vi "AlliGator Enter Reference Lifetime Dialog.vi"(8 "Error In":errorcluster, 11 "Input Message":string="Enter phase lifetime to use as refrence:") -> (0 "Error Out":errorcluster, 1 "Cancelled?":bool, 3 "Reference Lifetime":dbl[unit])   [LabVIEW 2021, in "AlliGator Phasor Graph.lvlib"]
doc: "Reference Lifetime dialog."
uses:
  AlliGator Phasor Graph.lvlib
panel:
  in  "Reference Lifetime":dbl[unit] min=0.0 format="%.3g"
  in  "Cancel":bool
  in  "OK":bool
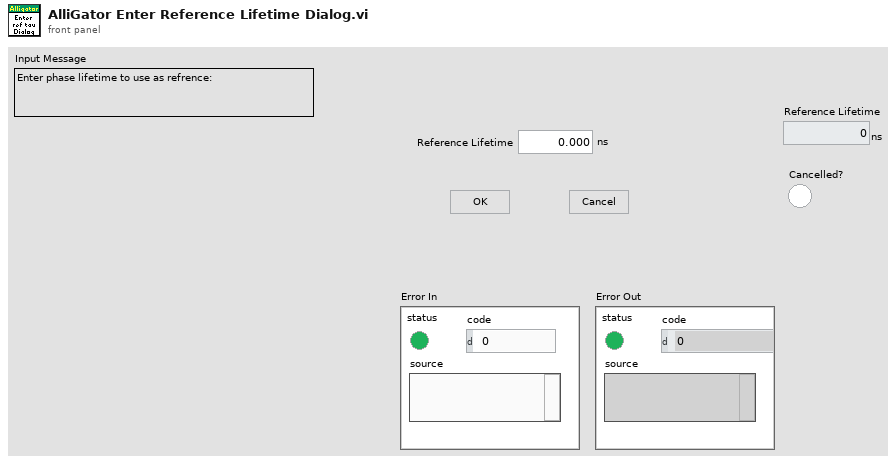
[diagram p1: front panel]
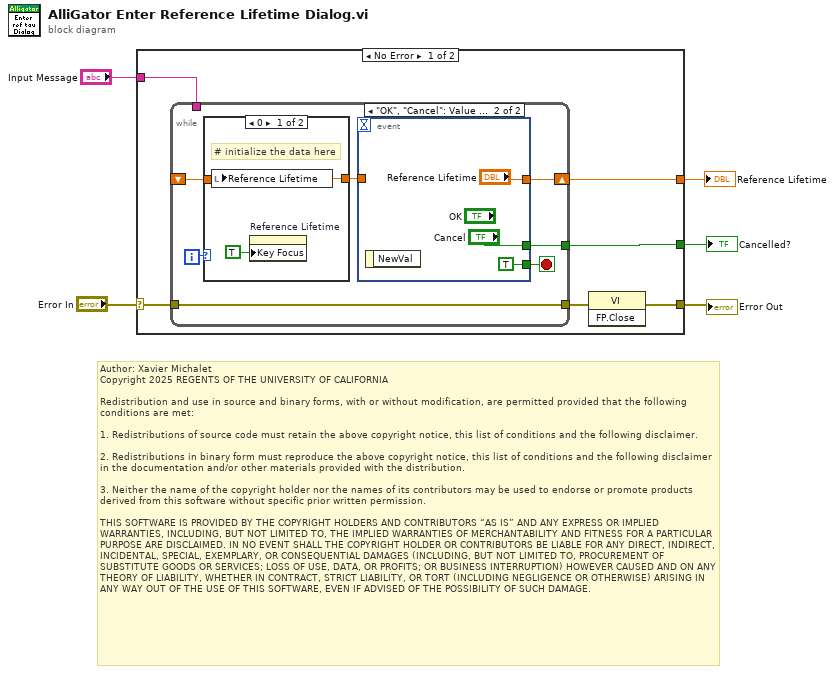
[diagram p0: block diagram]
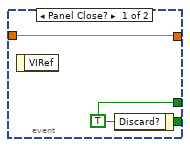
[diagram p3: hidden frame]
diagram:
  # "Author: Xavier Michalet\nCopyright 2025 REGENTS OF THE UNIVERSITY OF CALIFORNIA\n\nRedistribution and use in source and binary forms, with or without modification, are permitted provided that the following conditions are met:\n\n1. Redistributions of source code must retain the above copyright notice, this list of conditions and the following disclaimer.\n\n2. Redistributions in binary form must reproduce the above copyright notice, this list of conditions and the following disclaimer in the documentation and/or other materials provided with the distribution.\n\n3. Neither the name of the copyright holder nor the names of its contributors may be used to endorse or promote products derived from this software without specific prior written permission.\n\nTHIS SOFTWARE IS PROVIDED BY THE COPYRIGHT HOLDERS AND CONTRIBUTORS “AS IS” AND ANY EXPRESS OR IMPLIED WARRANTIES, INCLUDING, BUT NOT LIMITED TO, THE IMPLIED WARRANTIES OF MERCHANTABILITY AND FITNESS FOR A PARTICULAR PURPOSE ARE DISCLAIMED. IN NO EVENT SHALL THE COPYRIGHT HOLDER OR CONTRIBUTORS BE LIABLE FOR ANY DIRECT, INDIRECT, INCIDENTAL, SPECIAL, EXEMPLARY, OR CONSEQUENTIAL DAMAGES (INCLUDING, BUT NOT LIMITED TO, PROCUREMENT OF SUBSTITUTE GOODS OR SERVICES; LOSS OF USE, DATA, OR PROFITS; OR BUSINESS INTERRUPTION) HOWEVER CAUSED AND ON ANY THEORY OF LIABILITY, WHETHER IN CONTRACT, STRICT LIABILITY, OR TORT (INCLUDING NEGLIGENCE OR OTHERWISE) ARISING IN ANY WAY OUT OF THE USE OF THIS SOFTWARE, EVEN IF ADVISED OF THE POSSIBILITY OF SUCH DAMAGE."
  n1 = case shown="No Error" "Error In" {
    selector: "Error In" -> [w7 w27]
    tunnel: [w11 _] -> w5
    tunnel: [w10 _] -> w4
    tunnel: "Input Message" -> [w9 _]
    tunnel: [w8 w27] -> w1
    frame No Error {
      n2 = while {
        tunnel: [w17] -> w11
        shift-right: [w14] -> w10
        shift-left: _ -> [w15]
        tunnel: w9 -> [_]
        tunnel: w7 -> [w12]
        tunnel: [w12] -> w6
        i -> [w16]
        stop <- w18 stop-if-true
        n3 = case shown="0" w16 {
          tunnel: w15 -> [w20 w21]
          tunnel: [w20 w21] -> w13
          frame 0 {
            # "# initialize the data here"
            n4 = local write "Reference Lifetime"(w20) -> ()
            n5 = property on="Reference Lifetime" class="DigNum (strict)"("Key Focus"=TRUE) -> ()  [unwired: 2 in, 2 out]
          }
          frame 1, Default {
          }
        }
        n6 = event shown="[1] \"OK\", \"Cancel\": Value Change" {
          selector: _ -> [_ _]
          dyn-events: _ -> [_ _]
          timeout: _ -> [_ _]
          tunnel: [w23 TRUE ("Discard?")] -> w18
          tunnel: [w23 "Cancel"] -> w17
          tunnel: [w22 "Reference Lifetime"] -> w14
          tunnel: w13 -> [w22 _]
          event Panel Close? {
            w23 = TRUE ("Discard?")
            n7 = event-data() -> ()  [unwired: 1 in, 1 out]
            n8 = event-data("Discard?"=w23) -> ()  [unwired: 1 in, 1 out]
          }
          event "OK", "Cancel": Value Change {
            n9 = event-data() -> ()  [unwired: 1 in, 1 out]
          }
        }
      }
      n10 = invoke class="VI" method="FP.Close"(error in=w6) -> (error out=w8:errorcluster)  [unwired: 2 in, 2 out]
    }
    frame Error {
    }
  }
  "Reference Lifetime" <- w4
  "Cancelled?" <- w5
  "Error Out" <- w1
